vi "subQuantization.vi"(2 "input":dbl[](array[numeric]), 3 "parameter":T1) -> (0 "output":dbl[][](array[numeric]), 1 "n":i32)   [LabVIEW 2014]
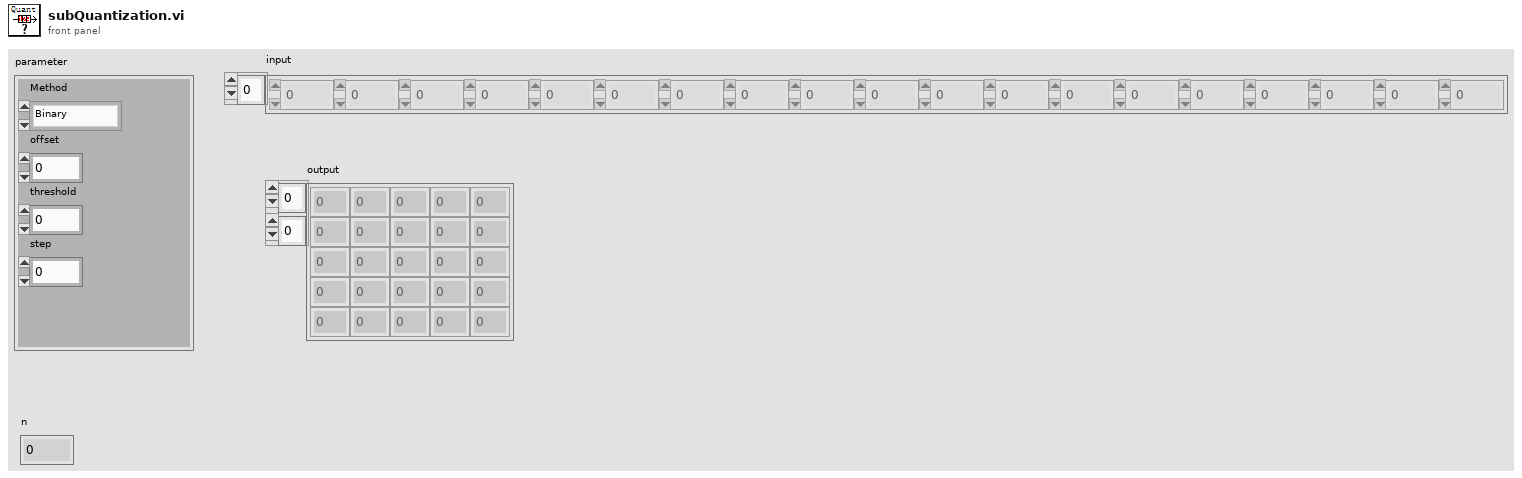
[diagram p1: front panel]
types:
  T1 = cluster{"Method":enum16{"Binary", "Uniform"}, "offset":i32, "threshold":dbl, "step":dbl}
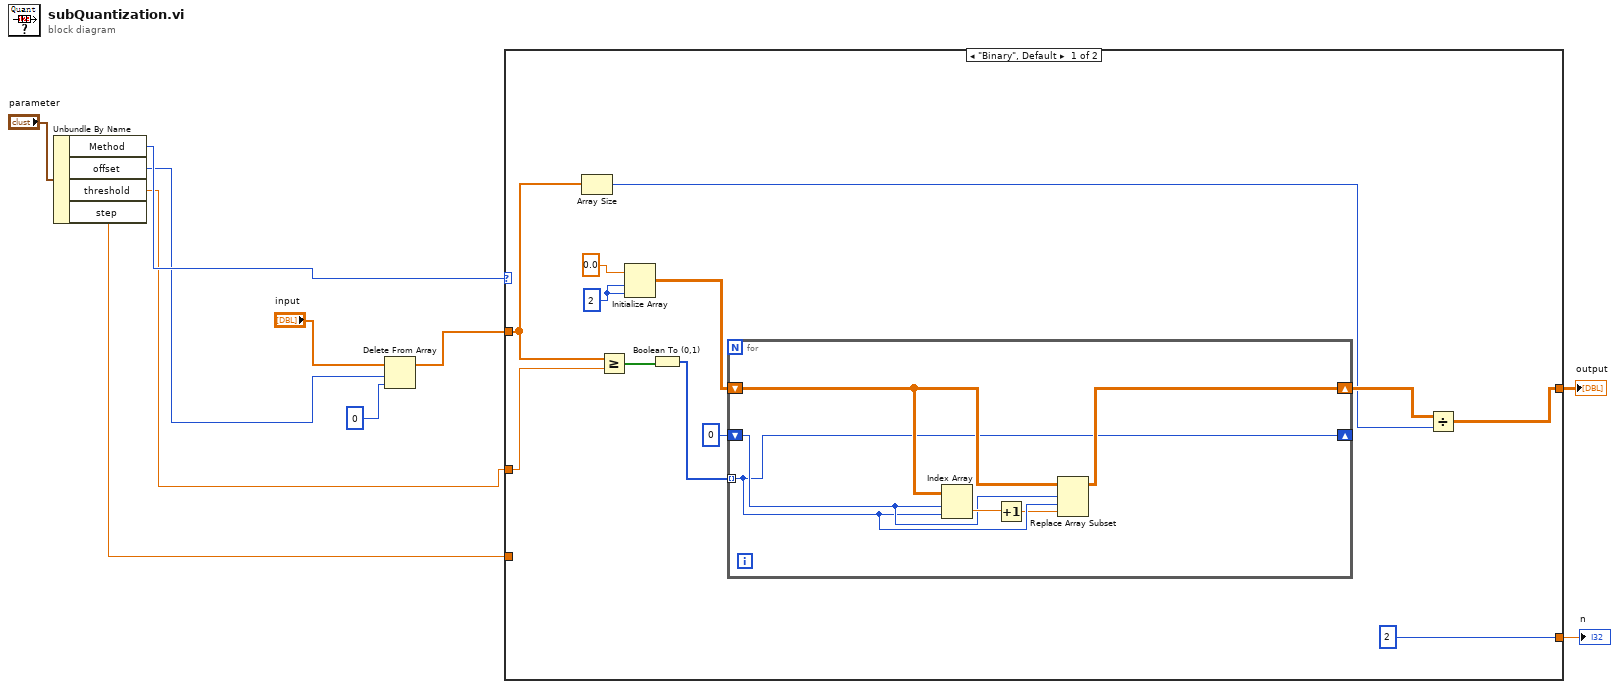
[diagram p0: block diagram]
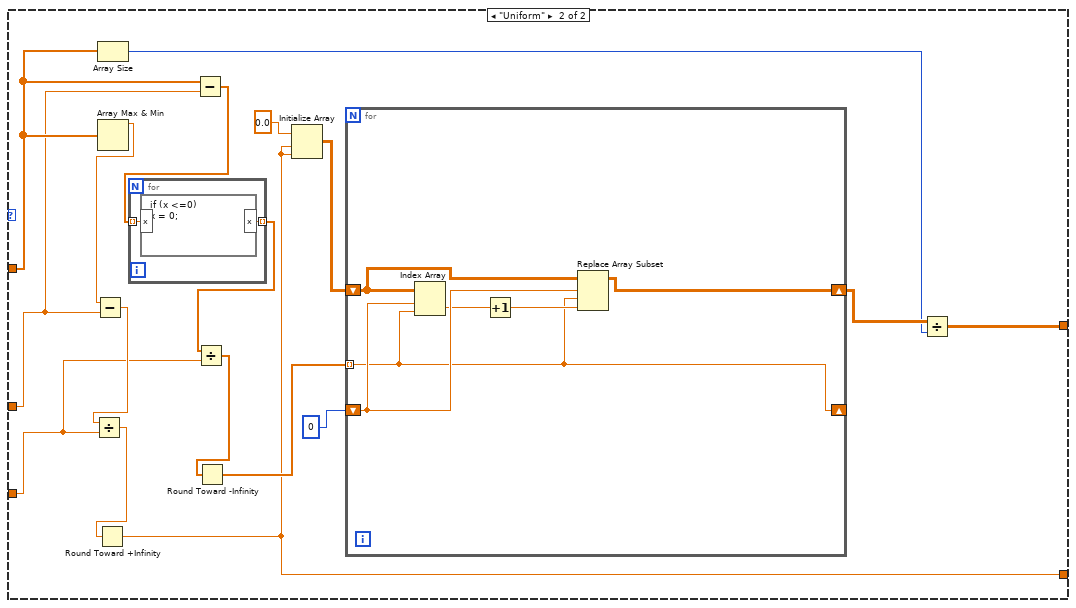
[diagram p2: hidden frame]
diagram:
  n1 = Unbundle By Name("parameter") -> ("Method"=w4:enum16{"Binary", "Uniform"}, "offset"=w3:i32, "threshold"=w2:dbl, "step"=w1:dbl)
  n2 = Delete From Array(array="input", length=w3, index=0) -> (array with subset deleted=w8:dbl[])  [unwired: 1 out]
  n3 = case shown="\"Binary\", Default" w4 {
    tunnel: w8 -> [w17 w41]
    tunnel: w2 -> [w22 w40]
    tunnel: [w12 w30] -> w7
    tunnel: w1 -> [_ w39]
    tunnel: [2 w29] -> w6
    frame "Binary", Default {
      w14 = 2 ("dimension size")
      n4 = Array Size(array=w17) -> (size(s)=w16:i32)
      n5 = Greater Or Equal?(x=w17, y=w22) -> (x >= y?=w21:bool[])
      n6 = Initialize Array(0.0 ("element"), w14, w14) -> (w19:dbl[][])
      n7 = Boolean To (0,1)(Boolean=w21) -> (0, 1=w13:i16[])
      n8 = for {
        tunnel: w13 -> [w24] mode=indexing
        shift-right: [w24] -> _
        shift-left: 0 -> [w25]
        shift-right: [w27] -> w18
        shift-left: w19 -> [w28]
        n9 = Index Array(array=w28, index (row)=w25, index (col)=w24) -> (element=w26:dbl)
        n10 = Increment(x=w26) -> (x+1=w23:dbl)
        n11 = Replace Array Subset(array=w28, new element=w23, index (row)=w25, index (col)=w24) -> (w27:dbl[][])
      }
      n12 = Divide(x=w18, y=w16) -> (x/y=w12:dbl[][])
    }
    frame "Uniform" {
      n13 = Array Size(array=w41) -> (size(s)=w31:i32)
      n14 = Array Max & Min(array=w41) -> (max value=w45:dbl)  [unwired: 3 out]
      n15 = Subtract(x=w45, y=w40) -> (x-y=w44:dbl)
      n16 = Divide(x=w44, y=w39) -> (x/y=w43:dbl)
      n17 = Round Toward +Infinity(x=w43) -> (ceil(x): smallest int >= x=w29:dbl)
      n18 = Subtract(x=w41, y=w40) -> (x-y=w34:dbl[])
      n19 = for {
        tunnel: w34 -> [w47] mode=indexing
        tunnel: [w46] -> w33 mode=indexing
        n20 = formula code="if (x <=0)\nx = 0;"("x"=w47) -> ("x"=w46:dbl)
      }
      n21 = Divide(x=w33, y=w39) -> (x/y=w38:dbl[])
      n22 = Round Toward -Infinity(1:w38) -> (0:w36:dbl[])
      n23 = Initialize Array(0.0 ("element"), w29, w29) -> (w37:dbl[][])
      n24 = for {
        tunnel: w36 -> [w48] mode=indexing
        shift-right: [w48] -> _
        shift-left: 0 -> [w52]
        shift-right: [w50] -> w32
        shift-left: w37 -> [w53]
        n25 = Index Array(array=w53, index (row)=w52, index (col)=w48) -> (element=w51:dbl)
        n26 = Increment(x=w51) -> (x+1=w49:dbl)
        n27 = Replace Array Subset(array=w53, new element=w49, index (row)=w52, index (col)=w48) -> (w50:dbl[][])
      }
      n28 = Divide(x=w32, y=w31) -> (x/y=w30:dbl[][])
    }
  }
  "output" <- w7
  "n" <- w6
